vi "calculateTimeStep.vi"(8 "error in (no error)":errorcluster, 11 "RampEvent in":refnum<class "RampEvent.lvclass">) -> (0 "error out":errorcluster, 1 "valueStep":dbl, 2 "timeStep":dbl, 3 "RampEvent out":refnum<class "RampEvent.lvclass">, 4 "number of Steps":i32)   [LabVIEW 2009, in "Tools.lvlib" / "Scripting.lvlib" / "RampEvent.lvclass"]
uses:
  RampEvent.lvclass
  RampEvent.lvclass/RampEvent.ctl
  ScriptEvent.lvclass
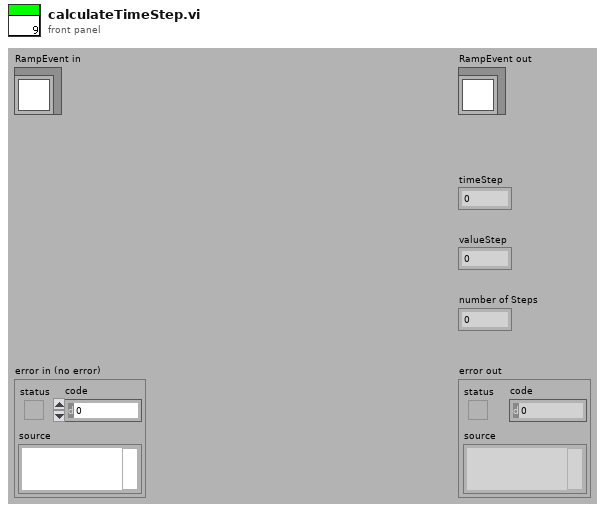
[diagram p1: front panel]
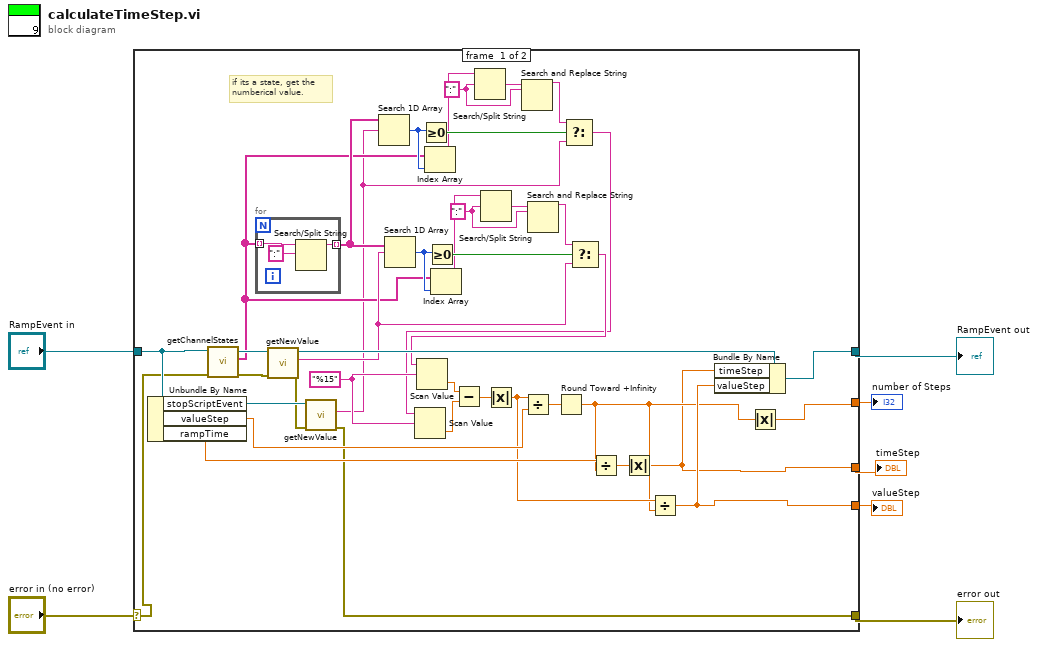
[diagram p0: block diagram]
diagram:
  n1 = case shown="No Error" "error in (no error)" {
    selector: "error in (no error)" -> [w32 w52]
    tunnel: [w35 w52] -> w6
    tunnel: [w36 w51] -> w4
    tunnel: "RampEvent in" -> [w34 w51]
    tunnel: [w9 _] -> w3
    tunnel: [w10 _] -> w2
    tunnel: [w12 _] -> w1
    frame #0 {
      w18 = ":"
      w26 = ":"
      w45 = "%15"
      # "if its a state, get the\nnumberical value."
      n2 = Unbundle By Name(w34) -> ("stopScriptEvent"=w47:refnum<class "ScriptEvent.lvclass">, "valueStep"=w41:dbl, "rampTime"=w40:dbl)
      n3 = call-dynamic "getChannelStates.vi"("error in (no error)"=w32, "ScriptEvent in"=w34) -> ("error out"=w31:errorcluster, "statesValues"=w15:string[], "ScriptEvent out"=w33:refnum<class "RampEvent.lvclass">)  [unwired: 7 in]
      n4 = for {
        tunnel: w15 -> [w50] mode=indexing
        tunnel: [w48] -> w16 mode=indexing
        n5 = Search/Split String(string=w50, search string/char (-)=":") -> (substring before match=w48:string)  [unwired: 1 in, 2 out]
      }
      n6 = call "getNewValue.vi"("error in (no error)"=w31, "ScriptEvent.lvclass in"=w33) -> ("error out"=w46:errorcluster, "newValue"=w24:string, "ScriptEvent.lvclass out"=w37:refnum<class "RampEvent.lvclass">)  [unwired: 7 in]
      n7 = call "getNewValue.vi"("error in (no error)"=w46, "ScriptEvent.lvclass in"=w47) -> ("error out"=w35:errorcluster, "newValue"=w14:string)  [unwired: 7 in, 1 out]
      n8 = Search 1D Array(1D array=w16, element=w14) -> (index of element=w22:i32)  [unwired: 1 in]
      n9 = Search 1D Array(1D array=w16, element=w24) -> (index of element=w30:i32)  [unwired: 1 in]
      n10 = Greater Or Equal To 0?(x=w22) -> (x >= 0?=w21:bool)
      n11 = Index Array(array=w15, index=w22) -> (element=w20:string)
      n12 = Greater Or Equal To 0?(x=w30) -> (x >= 0?=w29:bool)
      n13 = Index Array(array=w15, index=w30) -> (element=w28:string)
      n14 = Search/Split String(string=w20, search string/char (-)=w18) -> (match + rest of string=w19:string)  [unwired: 1 in, 2 out]
      n15 = Search/Split String(string=w28, search string/char (-)=w26) -> (match + rest of string=w27:string)  [unwired: 1 in, 2 out]
      n16 = Search and Replace String(input string=w19, search string=w18) -> (result string=w17:string)  [unwired: 6 in, 3 out]
      n17 = Search and Replace String(input string=w27, search string=w26) -> (result string=w25:string)  [unwired: 6 in, 3 out]
      n18 = Select(t=w17, s=w21, f=w14) -> (s? t:f=w13:string)
      n19 = Scan Value(string=w13, format string=w45) -> (value=w43:dbl)  [unwired: 1 in, 1 out]
      n20 = Select(t=w25, s=w29, f=w24) -> (s? t:f=w23:string)
      n21 = Scan Value(string=w23, format string=w45) -> (value=w44:dbl)  [unwired: 1 in, 1 out]
      n22 = Subtract(x=w44, y=w43) -> (x-y=w42:dbl)
      n23 = Absolute Value(x=w42) -> (abs(x)=w38:dbl)
      n24 = Divide(x=w38, y=w41) -> (x/y=w39:dbl)
      n25 = Round Toward +Infinity(x=w39) -> (ceil(x): smallest int >= x=w11:dbl)
      n26 = Divide(x=w40, y=w11) -> (x/y=w8:dbl)
      n27 = Absolute Value(x=w8) -> (abs(x)=w9:dbl)
      n28 = Divide(x=w38, y=w11) -> (x/y=w12:dbl)
      n29 = Bundle By Name(cluster=w37, "timeStep"=w9, "valueStep"=w12) -> (w36:refnum<class "RampEvent.lvclass">)
      n30 = Absolute Value(x=w11) -> (abs(x)=w10:dbl)
    }
    frame #1 {
    }
  }
  "error out" <- w6
  "RampEvent out" <- w4
  "timeStep" <- w3
  "number of Steps" <- w2
  "valueStep" <- w1
